vi "ForceTesting.vi"() -> ()   [LabVIEW 2021]
panel:
  out "Force (N)":dbl
  out "Force(N)":dynamicdata(graph)
  out "Force (g)":dbl
  out "Grams":dynamicdata(graph)
  out "Voltage":dbl
  out "Voltage":dynamicdata(graph)
  in  "stop (F)":bool
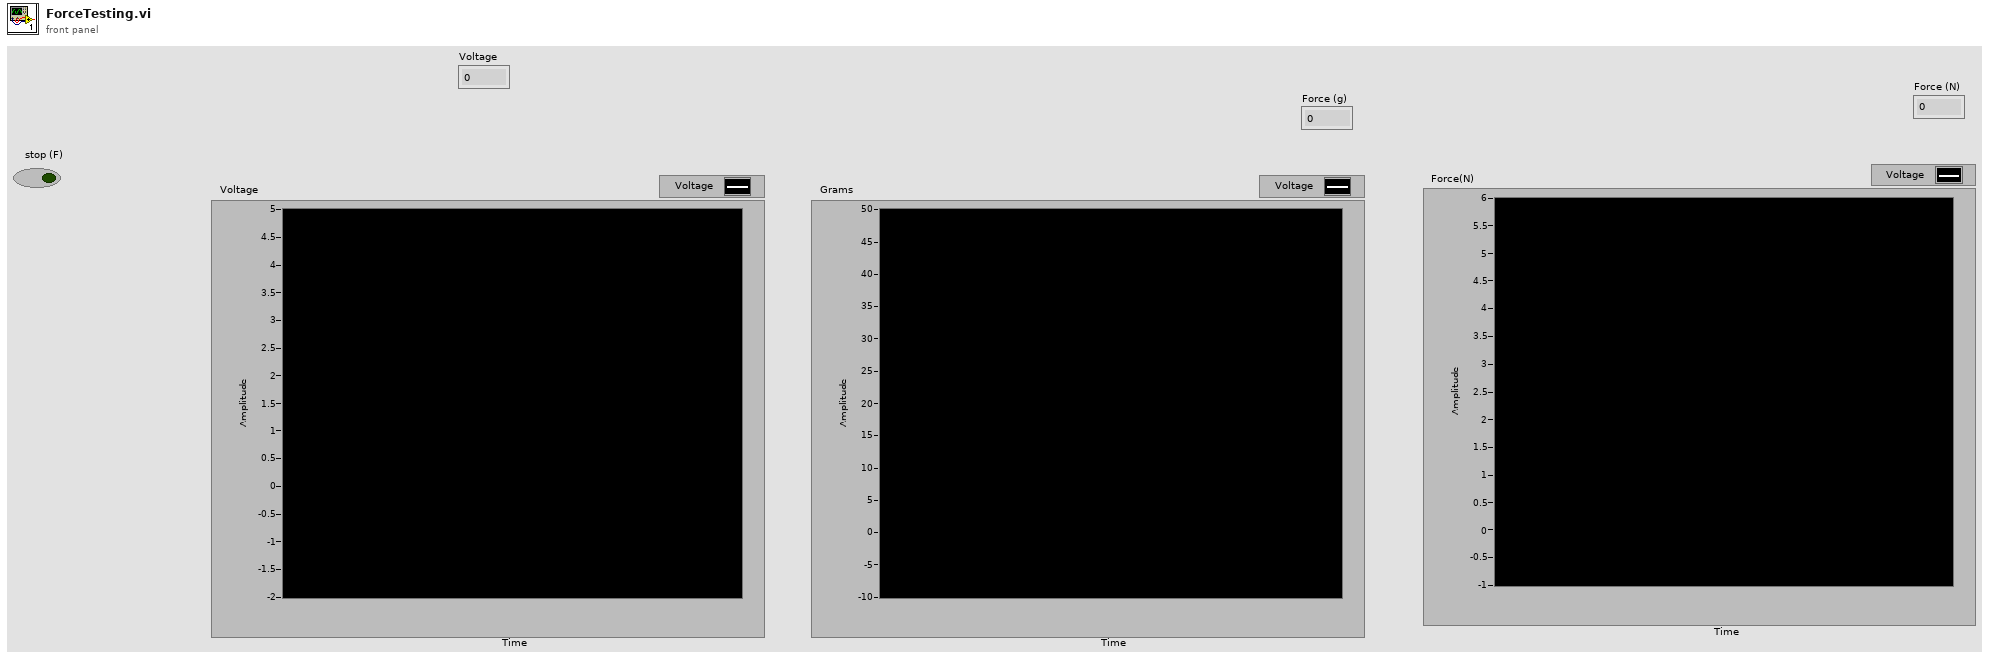
[diagram p1: front panel]
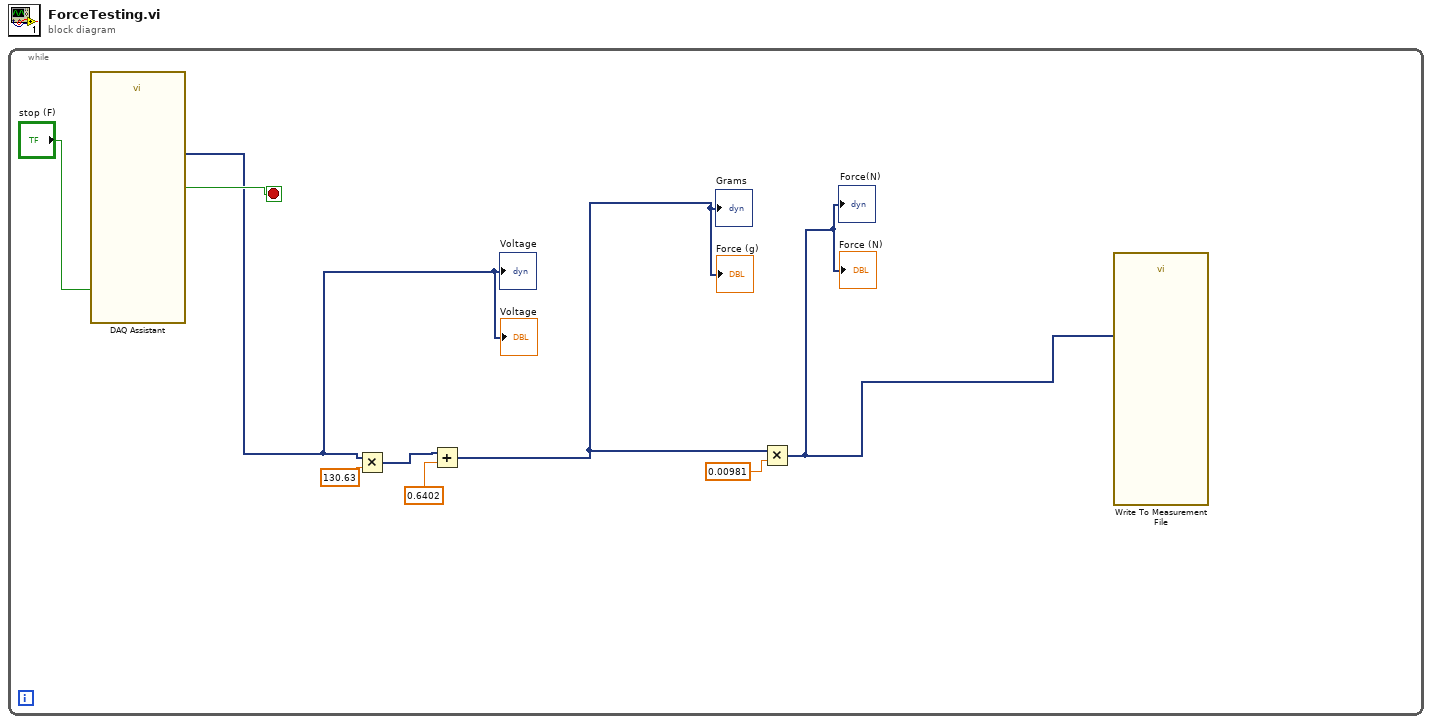
[diagram p0: block diagram]
diagram:
  n1 = while {
    stop <- w8 stop-if-true
    n2 = call "DAQ Assistant"("stop (F)"="stop (F)") -> ("data"=w4:dynamicdata, "stopped"=w8:bool)  [unwired: 15 in, 2 out]
    "Voltage" <- w4
    "Voltage" <- w4
    n3 = Multiply(x=w4, y=130.63) -> (x*y=w5:dynamicdata)
    n4 = Add(x=w5, y=0.6402) -> (x+y=w2:dynamicdata)
    "Grams" <- w2
    "Force (g)" <- w2
    n5 = Multiply(x=w2, y=0.00981) -> (x*y=w1:dynamicdata)
    "Force(N)" <- w1
    "Force (N)" <- w1
    n6 = call "Write To Measurement File"("Signals"=w1) -> ()  [unwired: 16 in, 3 out]
  }
